vi "PIM Display Key Array.vi"(4 "Conversion":enum16{"Cluster - HTML", "HTML - Cluster"}(ring), 6 "PIM Test Parameters":T1={"Stimulus"={"C1 Pwr dBm"=0.0, "C2 Pwr dBm"=0.0, "Power Units"=enum."dBm", "Meas Type"=enum."Time", "C1 Freq MHz"=0.0, "C2 Freq MHz"=0.0, "Swept Freq Step"=0}, "Measure"={"IM Order"=0, "Direction"=0, "Averaging"=1, "ALC ON?"=TRUE, "Peak Hold?"=TRUE, "Peak last N"=1, "Ref Level dBm"=-100.0, "Ref Units"=enum."dBm", "Num Samples"=1, "Sample units"=enum."Sample(s)", "Update Rate (s)"=0.0, "DUT PORT"=enum."Port 1", "Percent (%)"=100}, "Display"={"Power Scale"={"yRange_min"=0, "yRange_max"=0}, "xRange_span"=5}} {"Stimulus"."Swept Freq Step" items=[".2", ".4", "1.0", "2.0"]; "Measure"."Averaging" items=["None", "Minimum", "Normal", "High", "Maximum"]; "Measure"."Direction" items=["Reverse", "Forward", "Auxiliary"]; "Measure"."IM Order" items=["3rd", "5th", "7th", "9th", "11th", "13th", "15th", "17th", "19th", "21st", "23rd", "25th", "27th", "29th", "31st", "33rd"]}, 7 "Key Array In":T11) -> (1 "PIM Test Parameters (out)":T1={"Stimulus"={"C1 Pwr dBm"=0.0, "C2 Pwr dBm"=0.0, "Power Units"=enum."dBm", "Meas Type"=enum."Time", "C1 Freq MHz"=0.0, "C2 Freq MHz"=0.0, "Swept Freq Step"=0}, "Measure"={"IM Order"=0, "Direction"=0, "Averaging"=1, "ALC ON?"=TRUE, "Peak Hold?"=TRUE, "Peak last N"=1, "Ref Level dBm"=-100.0, "Ref Units"=enum."dBm", "Num Samples"=1, "Sample units"=enum."Sample(s)", "Update Rate (s)"=0.0, "DUT PORT"=enum."Port 1", "Percent (%)"=100}, "Display"={"Power Scale"={"yRange_min"=0, "yRange_max"=0}, "xRange_span"=5}} {"Stimulus"."Swept Freq Step" items=[".2", ".4", "1.0", "2.0"]; "Measure"."Averaging" items=["None", "Minimum", "Normal", "High", "Maximum"]; "Measure"."Direction" items=["Reverse", "Forward", "Auxiliary"]; "Measure"."IM Order" items=["3rd", "5th", "7th", "9th", "11th", "13th", "15th", "17th", "19th", "21st", "23rd", "25th", "27th", "29th", "31st", "33rd"]}, 2 "Key Array Out":T11)   [LabVIEW 2011]
uses:
  ITK/utils/keyedarr.llb/Keyed Array.ctl
  TypeDefs/PIM Test Parameters.ctl
  TypeDefs/PIM Stimulus Parameters.ctl
  BPIMCore/HW IO/PIM Sweep Step Size.ctl
  TypeDefs/PIM Measurement Parameters.ctl
  BPIMCore/HW IO/IMOrder.ctl
  BPIMCore/HW IO/MeasMode.ctl
  BPIMCore/HW IO/HW Averaging.ctl
  TypeDefs/PIM Meas Units.ctl
  BPIMCore/HW IO/DUTport.ctl
  TypeDefs/PIM Display Parameters.ctl
  ITK/utils/strutil.llb/Case Matching.ctl
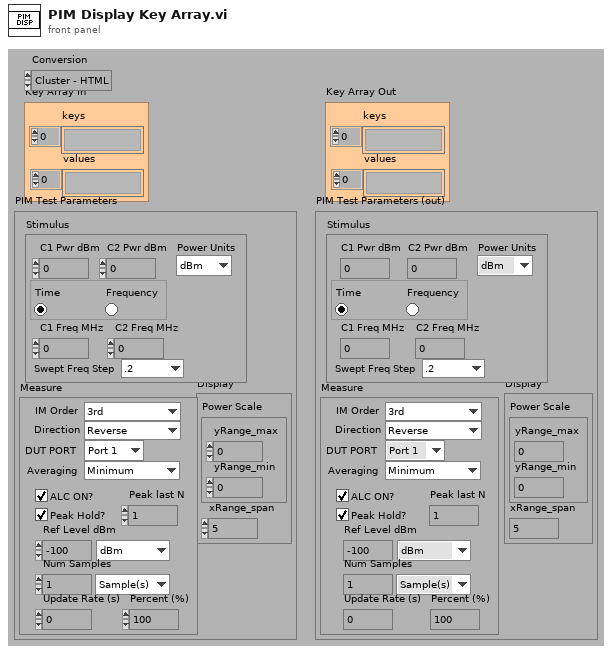
[diagram p1: front panel]
types:
  T1 = typedef "PIM Test Parameters.ctl" = cluster{"Stimulus":T2, "Measure":T4, "Display":T10}
  T2 = typedef "PIM Stimulus Parameters.ctl" = cluster{"C1 Pwr dBm":dbl, "C2 Pwr dBm":dbl, "Power Units":enum16{"dBm", "Watts"}, "Meas Type":enum32{"Time", "Frequency"}, "C1 Freq MHz":dbl, "C2 Freq MHz":dbl, "Swept Freq Step":T3}
  T3 = typedef "PIM Sweep Step Size.ctl" = u16
  T4 = typedef "PIM Measurement Parameters.ctl" = cluster{"IM Order":T5, "Direction":T6, "Averaging":T7, "ALC ON?":bool, "Peak Hold?":bool, "Peak last N":u32, "Ref Level dBm":dbl, "Ref Units":enum16{"dBm", "dBc"}, "Num Samples":u32, "Sample units":T8, "Update Rate (s)":dbl, "DUT PORT":T9, "Percent (%)":u8}
  T5 = typedef "IMOrder.ctl" = u8
  T6 = typedef "MeasMode.ctl" = u16
  T7 = typedef "HW Averaging.ctl" = u16
  T8 = typedef "PIM Meas Units.ctl" = enum16{"Sample(s)", "Second(s)", "Sweep(s)"}
  T9 = typedef "DUTport.ctl" = enum16{"Port 1", "Port 2"}
  T10 = typedef "PIM Display Parameters.ctl" = cluster{"Power Scale":cluster{"yRange_min":i32, "yRange_max":i32}, "xRange_span":u32}
  T11 = typedef "Keyed Array.ctl" = cluster{"keys":string[], "values":string[]}
  T12 = typedef "Case Matching.ctl" = enum16{"a != A", "a == A", "system"}
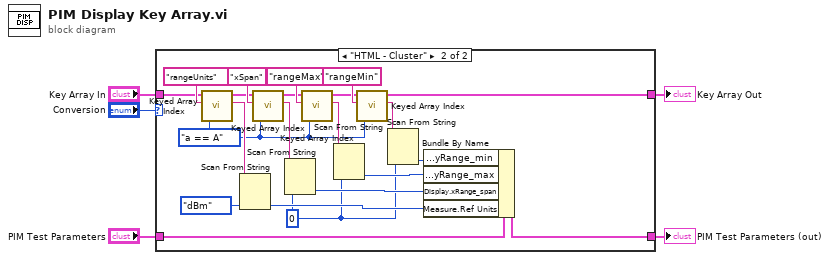
[diagram p0: block diagram]
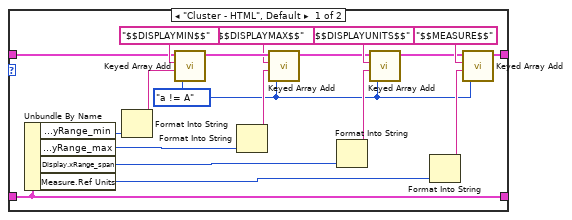
[diagram p2: hidden frame]
diagram:
  n1 = case shown="\"HTML - Cluster\"" "Conversion" {
    tunnel: "Key Array In" -> [w21 w30]
    tunnel: "PIM Test Parameters" -> [w8 w46]
    tunnel: [w7 w31] -> w3
    tunnel: [w8 w45] -> w2
    frame "Cluster - HTML", Default {
      w6 = Case_Matching."a != A" ("case matching (sensitive)")
      n2 = Unbundle By Name(w8) -> ("Display.Power Scale.yRange_min"=w16:i32, "Display.Power Scale.yRange_max"=w14:i32, "Display.xRange_span"=w12:u32, "Measure.Ref Units"=w9:enum16{"dBm", "dBc"})
      n3 = Format Into String(w16) -> (resulting string=w15:string)  [unwired: 3 in, 1 out]
      n4 = call "Keyed Array Add.vi"("case matching (sensitive)"=w6, "value"=w15, "key"="$$DISPLAYMIN$$", "array in"=w21) -> ("array out"=w24:T11)  [unwired: 3 out]
      n5 = Format Into String(w14) -> (resulting string=w13:string)  [unwired: 3 in, 1 out]
      n6 = call "Keyed Array Add.vi"("case matching (sensitive)"=w6, "value"=w13, "key"="$$DISPLAYMAX$$", "array in"=w24) -> ("array out"=w17:T11)  [unwired: 3 out]
      n7 = Format Into String(w12) -> (resulting string=w11:string)  [unwired: 3 in, 1 out]
      n8 = call "Keyed Array Add.vi"("case matching (sensitive)"=w6, "value"=w11, "key"="$$DISPLAYUNITS$$", "array in"=w17) -> ("array out"=w19:T11)  [unwired: 3 out]
      n9 = Format Into String(w9) -> (resulting string=w10:string)  [unwired: 3 in, 1 out]
      n10 = call "Keyed Array Add.vi"("case matching (sensitive)"=w6, "value"=w10, "key"="$$MEASURE$$", "array in"=w19) -> ("array out"=w7:T11)  [unwired: 3 out]
    }
    frame "HTML - Cluster" {
      w25 = 0 ("Display.Power Scale.yRange_min")
      w26 = Case_Matching."a == A" ("case matching (sensitive)")
      n11 = call "Keyed Array Index.vi"("case matching (sensitive)"=w26, "key"="rangeUnits", "array in"=w30) -> ("value"=w29:string, "duplicate array"=w32:T11)  [unwired: 1 in, 2 out]
      n12 = Scan From String(input string=w29, default 1=enum16{"dBm", "dBc"}."dBm" ("Measure.Ref Units")) -> (output 1=w27:enum16{"dBm", "dBc"})  [unwired: 3 in, 3 out]
      n13 = call "Keyed Array Index.vi"("case matching (sensitive)"=w26, "key"="xSpan", "array in"=w32) -> ("value"=w35:string, "duplicate array"=w36:T11)  [unwired: 1 in, 2 out]
      n14 = Scan From String(input string=w35, default 1=w25) -> (output 1=w34:i32)  [unwired: 3 in, 3 out]
      n15 = call "Keyed Array Index.vi"("case matching (sensitive)"=w26, "key"="rangeMax", "array in"=w36) -> ("value"=w39:string, "duplicate array"=w40:T11)  [unwired: 1 in, 2 out]
      n16 = Scan From String(input string=w39, default 1=w25) -> (output 1=w38:i32)  [unwired: 3 in, 3 out]
      n17 = call "Keyed Array Index.vi"("case matching (sensitive)"=w26, "key"="rangeMin", "array in"=w40) -> ("value"=w43:string, "duplicate array"=w31:T11)  [unwired: 1 in, 2 out]
      n18 = Scan From String(input string=w43, default 1=w25) -> (output 1=w44:i32)  [unwired: 3 in, 3 out]
      n19 = Bundle By Name(cluster=w46, "Display.Power Scale.yRange_min"=w44, "Display.Power Scale.yRange_max"=w38, "Display.xRange_span"=w34, "Measure.Ref Units"=w27) -> (w45:T1)
    }
  }
  "Key Array Out" <- w3
  "PIM Test Parameters (out)" <- w2
